vi "Clear Stack.vi"(7 "Keep Base Frame":bool=TRUE, 8 "error in (no error)":errorcluster, 11 "gScript Interpreter in":refnum<class "gScript Interpreter.lvclass">) -> (0 "error out":errorcluster, 3 "gScript Interpreter out":refnum<class "gScript Interpreter.lvclass">)   [LabVIEW 2017, in "gScript Interpreter.lvclass"]
uses:
  gScript Interpreter.lvclass
  gScript Interpreter.lvclass/gScript Interpreter.ctl
  Type Definitions/Stack Frame.ctl
  Type Definitions/Variable Table.ctl
  Type Definitions/Variable.ctl
  Type Definitions/Memory Cell.ctl
  Type Definitions/Memory Cell Type Enum.ctl
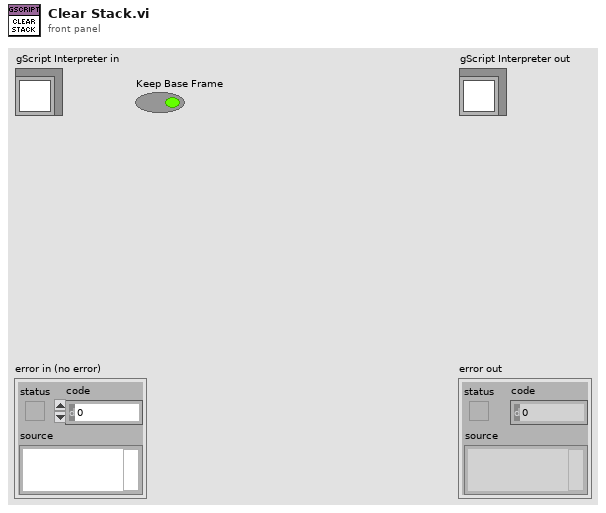
[diagram p1: front panel]
types:
  T1 = typedef "Stack Frame.ctl" = cluster{"Variable Table":T2, "Return Pointer":i32, "Return Bindings":string[]}
  T2 = typedef "Variable Table.ctl" = T3[]
  T3 = typedef "Variable.ctl" = cluster{"Variable Name":string, "Memory Cell":T4}
  T4 = typedef "Memory Cell.ctl" = cluster{"type":T5, "x":dbl, "y":dbl, "z":dbl, "w":dbl}
  T5 = typedef "Memory Cell Type Enum.ctl" = enum16{"integer", "float", "vector", "rotation"}
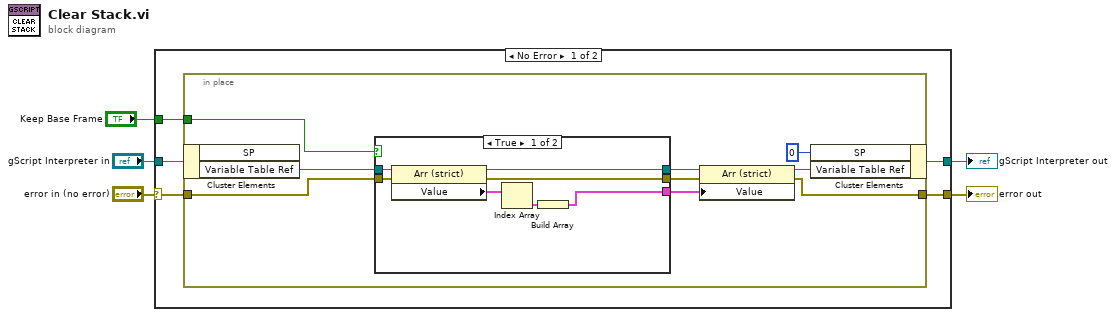
[diagram p0: block diagram]
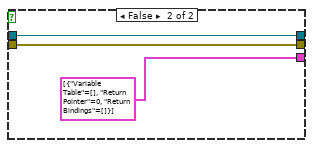
[diagram p2: hidden frame]
diagram:
  n1 = case shown="No Error" "error in (no error)" {
    selector: "error in (no error)" -> [w9 w31]
    tunnel: [w8 w31] -> w4
    tunnel: [w7 w30] -> w2
    tunnel: "gScript Interpreter in" -> [w10 w30]
    tunnel: "Keep Base Frame" -> [w6 _]
    frame No Error {
      n2 = in-place {
        in-place-border: w9 -> [w12]
        in-place-border: [w16] -> w8
        in-place-border: w6 -> [w13]
        n3 = in-place-cluster #1(w10) -> ("Variable Table Ref"=w15:refnum<vi>)  [unwired: 1 out]
        n4 = case shown="True" w13 {
          tunnel: [w20 T1[] [{"Variable Table"=[], "Return Pointer"=0, "Return Bindings"=[]}] ("Value")] -> w18
          tunnel: w15 -> [w26 w28]
          tunnel: [w24 w28] -> w14
          tunnel: w12 -> [w25 w27]
          tunnel: [w23 w27] -> w11
          frame True {
            n5 = property class="Arr (strict)"(reference=w26, error in=w25) -> (reference out=w24:refnum<vi>, error out=w23:errorcluster, "Value"=w22:T1[])
            n6 = Index Array(array=w22) -> (element=w21:T1)  [unwired: 1 in]
            n7 = Build Array(w21) -> (w20:T1[])
          }
          frame False {
          }
        }
        n8 = property class="Arr (strict)"(reference=w14, error in=w11, "Value"=w18) -> (reference out=w17:refnum<vi>, error out=w16:errorcluster)
        n9 = in-place-cluster #1("SP"=0, "Variable Table Ref"=w17) -> (w7:refnum<class "gScript Interpreter.lvclass">)
      }
    }
    frame Error {
    }
  }
  "error out" <- w4
  "gScript Interpreter out" <- w2
